vi "10-Tap 8-bit Camera without DRAM (FPGA-SIM).vi"() -> ()   [LabVIEW 2013]
doc: "This is the FPGA VI for the 10-Tap 8-Bit Camera with DRAM example. This example demonstrates how to acquire images from a 10-tap, 8-bit, extended configuration, Camera Link camera and transfer the images to the host. This example supports area scan and line scan cameras for both continuous and finite acquisitions.\n\nThis example also demonstrates the use of DRAM as a frame buffer for very high speed acquisitions. Data packing and flow-control are also employed to maximize use of the available DRAM and FIFOs in terms of both memory space and performance.\n\nAdditionally, the example demonstrates the serial server, which allows third-party camera configuration utilities to communicate with the camera using the Camera Link serial interface while this VI is running."
uses:
  Common/CL Signal Mapping.ctl
  Common/CL Configuration.ctl
  FPGA/Sector/Accumulate/Sector Parameter Cluster.ctl
  <vilib>/Platform/TimedLoop/XDataNode/timing_clust.ctl
  <vilib>/Platform/TimedLoop/XDataNode/nitl_modes.ctl
  <vilib>/Platform/TimedLoop/XDataNode/wakeup.ctl
  <vilib>/rvi/Emulation/niFpgaSctlEmulationGetInTimedLoop.vi
  <vilib>/rvi/Emulation/niFpgaEmulationReportErrorSimple.vi
  <vilib>/rvi/Emulation/niFpgaGetClockAttributes.vi
  <vilib>/rvi/Emulation/niFpgaCriticalErrorInLSC.vi
  <vilib>/rvi/FIFO/Fifo_Resource/nirvififoEmulationGetNumberOfElementsToWriteFpgaImpl.vi
  <vilib>/rvi/DataTransferAndStorage/Container/Common/niFpgaContainerGetUniqueNameForEmu.vi
  <vilib>/rvi/interface/RandomDataEmulation/nirviRandomDataFPGAFIFO.vi
  <vilib>/rvi/interface/RandomDataEmulation/niFpgaRandomDataHandleErrors.vi
  <vilib>/rvi/FIFO/Fifo_Resource/nirvififoEmulationWriteFpgaImpl.vi
  <vilib>/rvi/FIFO/Fifo_Resource/nirvififoEmulationGetNumberOfElementsToReadFpgaImpl.vi
  <vilib>/rvi/FIFO/Fifo_Resource/nirvififoEmulationReadFpgaImpl.vi
  <vilib>/rvi/Emulation/niFpgaProcessEmulError.vi
  FPGA/Globals/Sector Parameter Global.vi
  FPGA/Globals/Pixel Location Global.vi
  FPGA/Globals/Accumulated Sector Intensity.vi
  <vilib>/Platform/TimedLoop/XDataNode/XDataNode.xnode
  <vilib>/rvi/DataTransferAndStorage/Container/XNode/niFpgaContainer.xnode
  <vilib>/rvi/FIFO/Fifo_Resource/nirvififoEmulationGetNumberOfElementsToWrite.vi
  <vilib>/rvi/interface/RandomDataEmulation/nirviRandomDataFpgaReadWriteTemplate.vi
  <vilib>/rvi/FIFO/Fifo_Resource/nirvififoEmulationWrite.vi
  <vilib>/rvi/FIFO/Fifo_Resource/nirvififoEmulationGetNumberOfElementsToRead.vi
  <vilib>/rvi/FIFO/Fifo_Resource/nirvififoEmulationRead.vi
  <vilib>/Platform/TimedLoop/XDataNode/XDNodeRunTimeDep.lvlib
  FPGA/Globals/Wing Square Wave Frequency Global.vi
panel:
  out "Left Sector Edge":u8
  out "Right Sector Edge":u8
  in  "Right Start Angle Duty Cycle":fxp<+,8,0>
  in  "Right End Angle Duty Cycle":fxp<+,8,0>
  in  "Left End Angle Duty Cycle":fxp<+,8,0>
  in  "Left Start Angle Duty Cycle":fxp<+,8,0>
  out "Number of Elements to Write Sector Grouping FIFO":u32
  out "Analysis Ticks":u32
  out "Target Sim TO":bool
  out "Cam Data Timeout":bool
  out "Sector FIFO Timeout":bool
  out "Host DMA Timeout":bool
  out "Number of Elements to Read Cam Data":u32
  out "Number of Elements to Write Host DMA":u32
  in  "Words per image":u32=1000
  in  "Y Resolution":u16=1000
  in  "X Resolution":u16=1000
  in  "[Average BG Intensity]":u8[](array[numeric])=[0, 0, 0, 0, 0, 0, 0, 0, 0, 0, 0, 0, 0, 0, 0, 0, 0, 0, 0, 0, 0, 0, 0, 0, 0, 0, 0, 0, 0, 0, 0, 0]
  in  "Sector Threshold":u8
  in  "# of Frames to Average":u8=1
  in  "Sector Parameters Right":T1={"Start Angle"=0.0, "End Angle"=0.4708251953125, "Inner Radius"=309, "Outter Radius"=405, "Hinge X"=685, "Hinge Y"=527, "NumWingSectors"=8}
  in  "Sector Parameters Left":T1={"Start Angle"=0.65740966796875, "End Angle"=0.99468994140625, "Inner Radius"=309, "Outter Radius"=405, "Hinge X"=464, "Hinge Y"=534, "NumWingSectors"=8}
  in  "CL Config.Configuration":T2=enum."Full"
  in  "CL Config.Signal Mapping":T3=enum."Basler 10-tap"
  in  "CL Config.Line Scan":bool
  in  "CL Config.DVAL Active High":bool=TRUE
  in  "CL Config.LVAL Active High":bool=TRUE
  in  "CL Config.FVAL Active High":bool=TRUE
  in  "CL Config.Spare Active High":bool=TRUE
  in  "Acq Control.Line Scan Height":u32
  in  "Acq Control.Frames To Acq":u32
  in  "Acq Control.Acquire":bool
  in  "Acq Control.Cancel Acq":bool
  in  "Acq Control.Ignore DVAL":bool
  in  "Acq Control.Initialize":bool
  out "Acq Status.Acq In Progress":bool
  out "Acq Status.Clocks Per Line":u32
  out "Acq Status.Frames Acq'd":u32
  out "Acq Status.Lines Per Frame":u32
  out "Acq Status.DMA Write Timeout":bool
  out "Acq Status.Initialized":bool
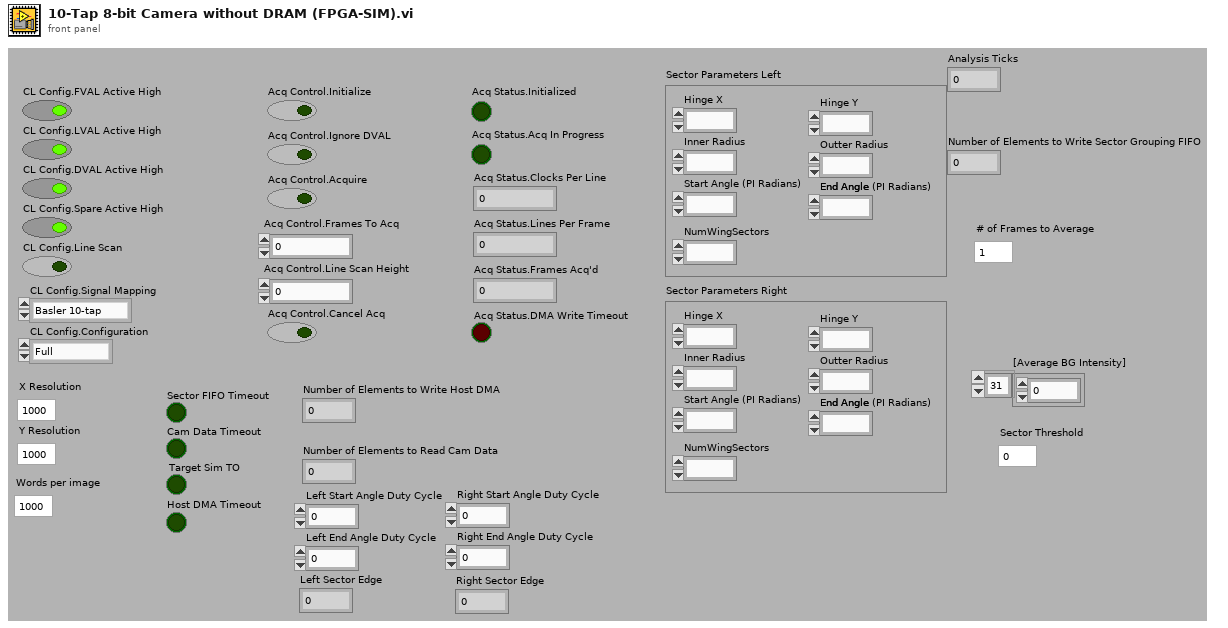
[diagram p1: front panel]
types:
  T1 = typedef "Sector Parameter Cluster.ctl" = cluster{"Start Angle":fxp<+/-,17,2>, "End Angle":fxp<+,17,3>, "Inner Radius":u16, "Outter Radius":u16, "Hinge X":u16, "Hinge Y":u16, "NumWingSectors":u8}
  T2 = typedef "CL Configuration.ctl" = enum8{"Base", "Medium", "Full"}
  T3 = typedef "CL Signal Mapping.ctl" = enum8{"Standard", "Basler 10-tap", "Vosskühler 10-tap"}
  T4 = typedef "XDNodeRunTimeDep.lvlib/timing_clust.ctl" = cluster{"Expected End [f-1]":u64, "Actual End [f-1]":u64, "Finished Late? [f-1]":bool, "Expected End [i-1]":u64, "Actual End [i-1]":u64, "Finished Late? [i-1]":bool, "Expected Start [i]":u64, "Actual Start [i]":u64, "Expected Start [f]":u64, "Actual Start [f]":u64, "Source Name":string, "Structure Name":string, "Period":i64, "Deadline":i64, "Offset":i64, "Start":i64, "Priority":i32, "Timeout":i32, "Mode":T5, "Wakeup Reason":T6, "Error":errorcluster, "Source Type":string, "Secondary Source Type":string, "Global End Time":u64, "Global Start Time":u64, "Frame Duration":u64, "Iteration Duration":u64, "Assigned CPU":i32, "I/O Scan Engine Mode":u32}
  T5 = typedef "XDNodeRunTimeDep.lvlib/nitl_modes.ctl" = enum32{"No Change", "Process missed periods, maintain original phase", "Discard missed periods, maintain original phase", "Process missed periods, ignore original phase", "Discard missed periods, ignore original phase"}
  T6 = typedef "XDNodeRunTimeDep.lvlib/wakeup.ctl" = enum32{"Normal", "Aborted", "Asynchronous wakeup", "Timing source error", "Timed loop error", "Timeout"}
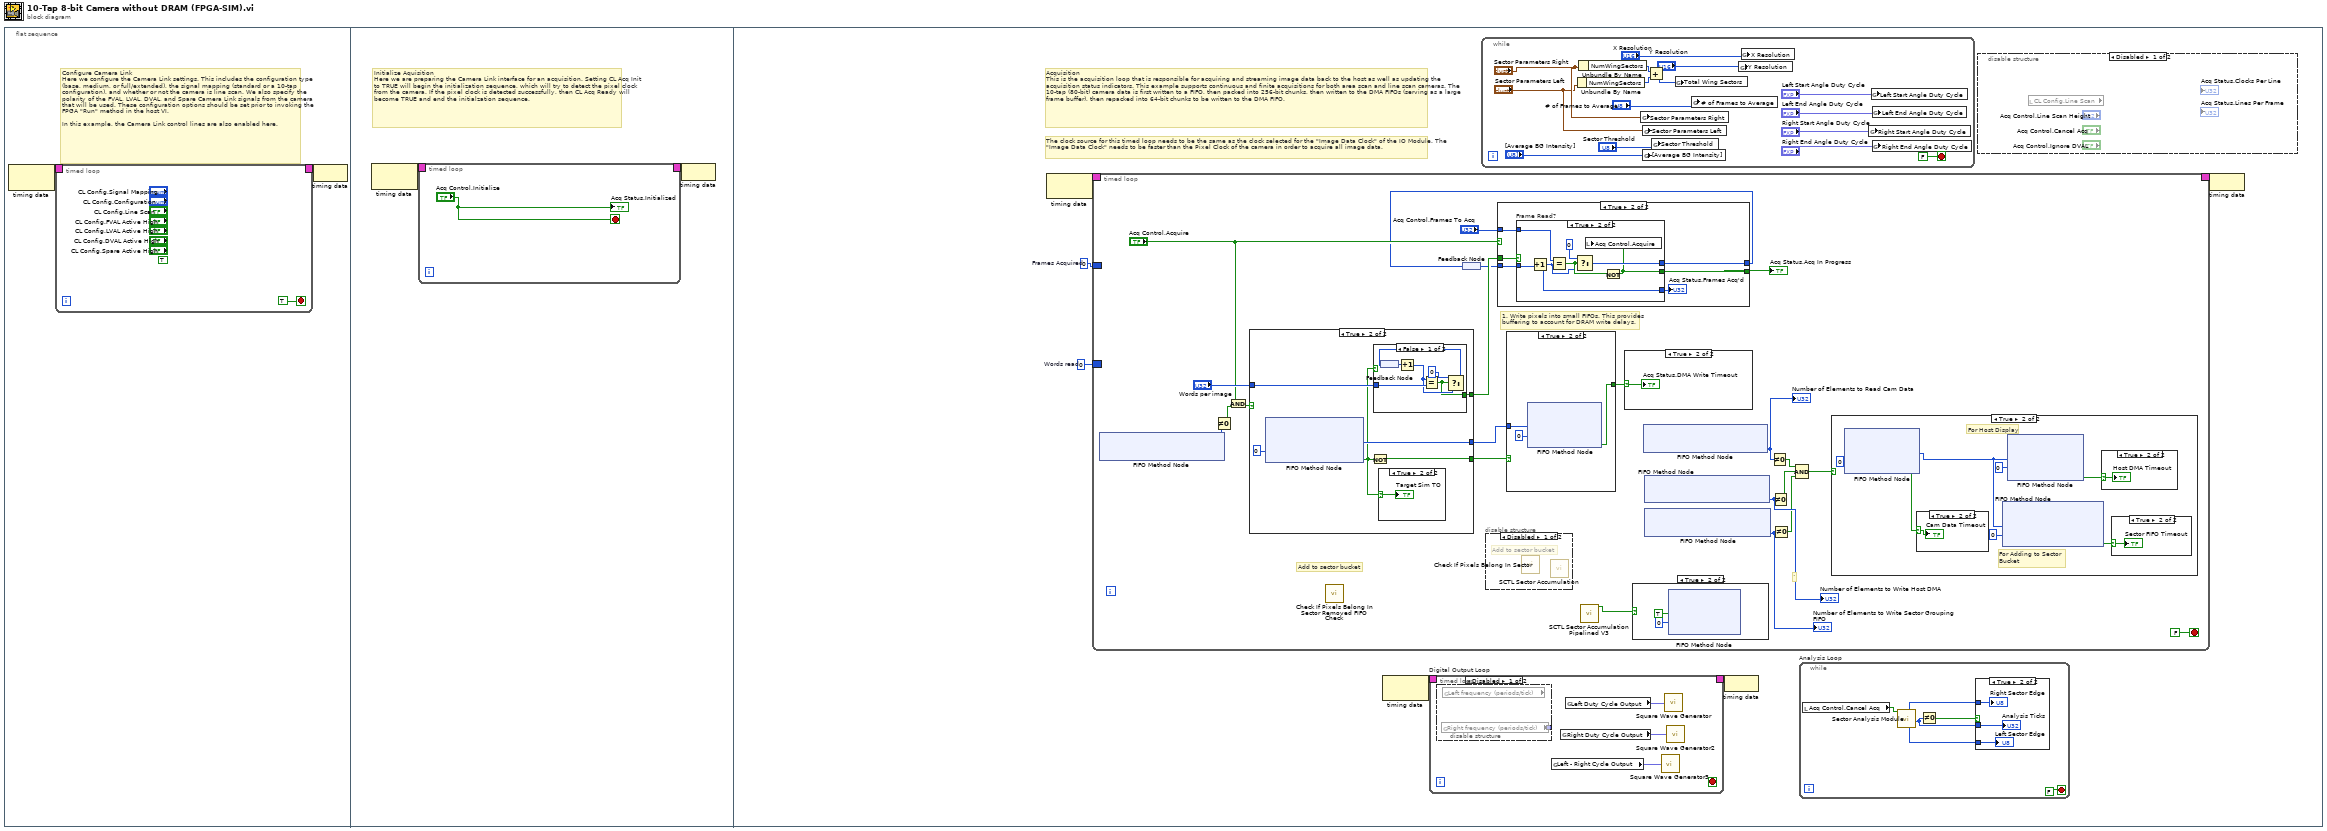
[diagram p0: block diagram]
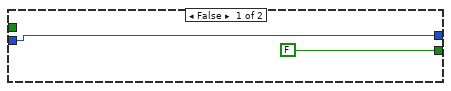
[diagram p8: hidden frame]
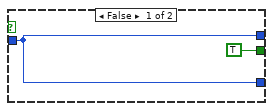
[diagram p9: hidden frame]
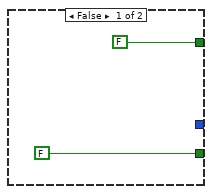
[diagram p10: hidden frame]
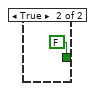
[diagram p12: hidden frame]
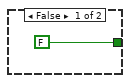
[diagram p17: hidden frame]
diagram:
  n1 = flat-sequence {
    frame #0 {
      # "Configure Camera Link\nHere we configure the Camera Link settings. This includes the configuration type (base, medium, or full/extended), the signal mapping (standard or a 10-tap configuration), and whether or not the camera is line scan. We also specify the polarity of the FVAL, LVAL, DVAL, and Spare Camera Link signals from the camera that will be used. These configuration options should be set prior to invoking the FPGA \"Run\" method in the host VI.\n\nIn this example, the Camera Link control lines are also enabled here."
      n2 = node-c288() -> (w2:T4)  [unwired: 1 in]
      n3 = timed-loop {
        timing: w2 -> [_]
        timing-out: [_] -> w1
        stop <- TRUE stop-if-true
        (unwired) TRUE ("IO Module\\CL Control Enable")
      }
      n4 = node-c288(w1) -> ()
    }
    frame #1 {
      # "Initialize Aquisition\nHere we are preparing the Camera Link interface for an acquisition. Setting CL Acq Init to TRUE will begin the initialization sequence, which will try to detect the pixel clock from the camera. If the pixel clock is detected successfully, then CL Acq Ready will become TRUE and end the initialzation sequence."
      n5 = node-c288() -> (w9:T4)  [unwired: 1 out]
      n6 = timed-loop {
        timing: w9 -> [_]
        timing-out: [_] -> w8
        stop <- "Acq Control.Initialize" stop-if-true
        "Acq Status.Initialized" <- "Acq Control.Initialize"
      }
      n7 = node-c288(w8) -> ()
    }
    frame #2 {
      w17 = u32 0  # Frames Acquired
      w18 = u32 0  # Words read
      # "The clock source for this timed loop needs to be the same as the clock selected for the \"Image Data Clock\" of the IO Module. The \"Image Data Clock\" needs to be faster than the Pixel Clock of the camera in order to acquire all image data."
      # "Acquisition\nThis is the acquisition loop that is responsible for acquiring and streaming image data back to the host as well as updating the acquisition status indicators. This example supports continuous and finite acquisitions for both area scan and line scan cameras. The 10-tap (80-bit) camera data is first written to a FIFO, then packed into 256-bit chunks, then written to the DMA FIFOs (serving as a large frame buffer), then repacked into 64-bit chunks to be written to the DMA FIFO."
      n8 = node-c288() -> (w20:T4)  [unwired: 1 in]
      n9 = timed-loop {
        timing: w20 -> [_]
        timing-out: [_] -> w19
        border: w18 -> [_]
        border: w17 -> [_]
        stop <- FALSE stop-if-true
        # "`"
        # "Add to sector bucket"
        # "1. Write pixels into small FIFOs. This provides\nbuffering to account for DRAM write delays."
        n10 = xnode ("FIFO Method Node")() -> ("Number of Elements to Write"=w53:u32)  [unwired: 1 in, 1 out]
        n11 = Not Equal To 0?(x=w53) -> (x != 0?=w52:bool)
        n12 = And(x="Acq Control.Acquire", y=w52) -> (x .and. y?=w60:bool)
        n13 = case shown="True" w60 {
          tunnel: [_ w92] -> w64
          tunnel: [FALSE w88] -> w62
          tunnel: "Words per image" -> [_ w90]
          tunnel: [FALSE w89] -> w49
          frame False {
          }
          frame True {
            n14 = xnode ("FIFO Method Node")("Timeout"=0) -> ("Element"=w92:u64, "Timed Out?"=w87:bool)  [unwired: 1 in, 1 out]
            n15 = Not(x=w87) -> (.not. x?=w88:bool)
            n16 = case shown="False" w87 {
              tunnel: w90 -> [w99 _]
              tunnel: [w94 FALSE] -> w89
              frame False {
                n17 = feedback #1() -> (w98:u32)
                n18 = Increment(x=w98) -> (x+1=w95:u32)
                n19 = Equal?(x=w95, y=w99) -> (x = y?=w94:bool)
                n20 = Select(t=u32 0 ("Acq Status.Frames Acq'd"), s=w94, f=w95) -> (s? t:f=w96:u32)
                n21 = feedback-in #1(w96) -> ()
              }
              frame True {
              }
            }
            n22 = case shown="True" w87 {
              selector: w87 -> [_ w93]
              frame False {
              }
              frame True {
                "Target Sim TO" <- w93
              }
            }
          }
        }
        n23 = call "Check If Pixels Belong In Sector Removed FIFO Check.vi"() -> ()  [unwired: 11 in, 1 out]
        n24 = feedback #2() -> (w48:u32)
        n25 = disable-structure shown="Disabled" {
          frame Disabled {
            # "Add to sector bucket"
            n26 = call "Check If Pixels Belong In Sector.vi"() -> ()  [unwired: 11 in, 1 out]
            n27 = call "SCTL Sector Accumulation.vi"() -> ()  [unwired: 11 in, 1 out]
          }
          frame Enabled {
          }
        }
        n28 = case shown="True" "Acq Control.Acquire" {
          tunnel: w49 -> [_ w75]
          tunnel: w48 -> [w69 w74]
          tunnel: "Acq Control.Frames To Acq" -> [_ w73]
          tunnel: [w69 w72] -> w46
          tunnel: [FALSE w71] -> w45
          frame False {
          }
          frame True {
            n29 = case "Frame Read?" shown="True" w75 {
              tunnel: w74 -> [w76 w84]
              tunnel: w73 -> [_ w83]
              tunnel: [w76 w81] -> w72
              tunnel: [TRUE w79] -> w71
              tunnel: [w76 w78] -> w70
              frame False {
              }
              frame True {
                n30 = Increment(x=w84) -> (x+1=w78:u32)
                n31 = Equal?(x=w83, y=w78) -> (x = y?=w80:bool)
                n32 = Select(t=u32 0 ("Frames Acquired"), s=w80, f=w78) -> (s? t:f=w81:u32)
                n33 = Not(x=w80) -> (.not. x?=w79:bool)
                n34 = local write "Acq Control.Acquire"(w79) -> ()
              }
            }
            "Acq Status.Frames Acq'd" <- w70
          }
        }
        "Acq Status.Acq In Progress" <- w45
        n35 = feedback-in #2(w46) -> ()
        n36 = case shown="True" w62 {
          tunnel: [FALSE ("Timed Out?") w113] -> w44
          tunnel: w64 -> [_ w114]
          frame False {
          }
          frame True {
            n37 = xnode ("FIFO Method Node")("Element"=w114, "Timeout"=0) -> ("Timed Out?"=w113:bool)  [unwired: 1 in, 1 out]
          }
        }
        n38 = call "SCTL Sector Accumulation Pipelined V3.vi"() -> ("New Data?"=w43:bool)  [unwired: 11 in]
        n39 = case shown="True" w44 {
          selector: w44 -> [_ w67]
          frame False {
          }
          frame True {
            "Acq Status.DMA Write Timeout" <- w67
          }
        }
        n40 = case shown="True" w43 {
          frame False {
          }
          frame True {
            n41 = xnode ("FIFO Method Node")("Element"=TRUE, "Timeout"=0) -> ()  [unwired: 1 in, 2 out]
          }
        }
        n42 = xnode ("FIFO Method Node")() -> ("Number of Elements to Read"=w55:u32)  [unwired: 1 in, 1 out]
        "Number of Elements to Read Cam Data" <- w55
        n43 = xnode ("FIFO Method Node")() -> ("Number of Elements to Write"=w58:u32)  [unwired: 1 in, 1 out]
        "Number of Elements to Write Host DMA" <- w58
        n44 = xnode ("FIFO Method Node")() -> ("Number of Elements to Write"=w57:u32)  [unwired: 1 in, 1 out]
        "Number of Elements to Write Sector Grouping FIFO" <- w57
        n45 = Not Equal To 0?(x=w55) -> (x != 0?=w54:bool)
        n46 = Not Equal To 0?(x=w58) -> (x != 0?=w59:bool)
        n47 = Not Equal To 0?(x=w57) -> (x != 0?=w56:bool)
        n48 = Compound Arithmetic op=AND(w54, w59, w56) -> (w61:bool)
        n49 = case shown="True" w61 {
          frame False {
          }
          frame True {
            # "For Adding to Sector \nBucket"
            # "For Host Display"
            n50 = xnode ("FIFO Method Node")("Timeout"=0) -> ("Element"=w105:u64, "Timed Out?"=w101:bool)  [unwired: 1 in, 1 out]
            n51 = case shown="True" w101 {
              selector: w101 -> [_ w108]
              frame False {
              }
              frame True {
                "Cam Data Timeout" <- w108
              }
            }
            n52 = xnode ("FIFO Method Node")("Element"=w105, "Timeout"=0) -> ("Timed Out?"=w103:bool)  [unwired: 1 in, 1 out]
            n53 = xnode ("FIFO Method Node")("Element"=w105, "Timeout"=0) -> ("Timed Out?"=w102:bool)  [unwired: 1 in, 1 out]
            n54 = case shown="True" w102 {
              selector: w102 -> [_ w109]
              frame False {
              }
              frame True {
                "Host DMA Timeout" <- w109
              }
            }
            n55 = case shown="True" w103 {
              selector: w103 -> [_ w110]
              frame False {
              }
              frame True {
                "Sector FIFO Timeout" <- w110
              }
            }
          }
        }
      }
      n56 = node-c288() -> (w16:T4)  [unwired: 1 in]
      n57 = timed-loop "Digital Output Loop" {
        timing: w16 -> [_]
        timing-out: [_] -> w15
        stop <- _ stop-if-true
        n58 = disable-structure shown="Disabled" {
          disable-tunnel: [w24 _] -> _
          frame Disabled {
            n59 = global read "Wing Square Wave Frequency Global.vi" "Right frequency (periods/tick)"() -> (w24:fxp<+,32,0>)
            n60 = global read "Wing Square Wave Frequency Global.vi" "Left frequency (periods/tick)"() -> ()  [unwired: 1 out]
          }
          frame Enabled {
          }
        }
        n61 = global read "Sector Parameter Global.vi" "Left - Right Cycle Output"() -> (w21:fxp<+,8,0>)
        n62 = global read "Sector Parameter Global.vi" "Right Duty Cycle Output"() -> (w22:fxp<+,8,0>)
        n63 = global read "Sector Parameter Global.vi" "Left Duty Cycle Output"() -> (w23:fxp<+,8,0>)
        n64 = call "Square Wave Generator3"("duty cycle (periods)"=w21) -> ()  [unwired: 14 in, 1 out]
        n65 = call "Square Wave Generator"("duty cycle (periods)"=w23) -> ()  [unwired: 14 in, 1 out]
        n66 = call "Square Wave Generator2"("duty cycle (periods)"=w22) -> ()  [unwired: 14 in, 1 out]
      }
      n67 = while {
        stop <- FALSE stop-if-true
        n68 = Unbundle By Name("Sector Parameters Left") -> ("NumWingSectors"=w131:u8)
        n69 = Unbundle By Name("Sector Parameters Right") -> ("NumWingSectors"=w132:u8)
        n70 = global write "Sector Parameter Global.vi" "Sector Parameters Right"("Sector Parameters Right") -> ()
        n71 = global write "Sector Parameter Global.vi" "Sector Parameters Left"("Sector Parameters Left") -> ()
        n72 = global write "Sector Parameter Global.vi" "[Average BG Intensity]"("[Average BG Intensity]") -> ()
        n73 = Add(x=w132, y=w131) -> (x+y=w130:u8)
        n74 = global write "Sector Parameter Global.vi" "Sector Threshold"("Sector Threshold") -> ()
        n75 = global write "Accumulated Sector Intensity.vi" "Total Wing Sectors"(w130) -> ()
        n76 = global write "Pixel Location Global.vi" "# of Frames to Average"("# of Frames to Average") -> ()
        n77 = global write "Pixel Location Global.vi" "Y Resolution"("Y Resolution") -> ()
        n78 = global write "Pixel Location Global.vi" "X Resolution"("X Resolution") -> ()
        n79 = global write "Sector Parameter Global.vi" "Right Start Angle Duty Cycle"("Right Start Angle Duty Cycle") -> ()
        n80 = global write "Sector Parameter Global.vi" "Left Start Angle Duty Cycle"("Left Start Angle Duty Cycle") -> ()
        n81 = global write "Sector Parameter Global.vi" "Left End Angle Duty Cycle"("Left End Angle Duty Cycle") -> ()
        n82 = global write "Sector Parameter Global.vi" "Right End Angle Duty Cycle"("Right End Angle Duty Cycle") -> ()
      }
      n83 = node-c288(w15) -> ()
      n84 = while "Analysis Loop" {
        stop <- FALSE stop-if-true
        n85 = local read "Acq Control.Cancel Acq"() -> (w38:bool)
        n86 = call "Sector Analysis Module.vi"("Canceled?"=w38) -> ("Analysis Ticks"=w37:u32, "Left Sector Edge"=w34:u8, "Right Sector Edge"=w35:u8)  [unwired: 6 in, 2 out]
        n87 = Not Equal To 0?(x=w37) -> (x != 0?=w36:bool)
        n88 = case shown="True" w36 {
          tunnel: w37 -> [_ w42]
          tunnel: w35 -> [_ w41]
          tunnel: w34 -> [_ w40]
          frame False {
          }
          frame True {
            "Analysis Ticks" <- w42
            "Right Sector Edge" <- w41
            "Left Sector Edge" <- w40
          }
        }
      }
      n89 = disable-structure shown="Disabled" {
        frame Disabled {
          n90 = local read "CL Config.Line Scan"() -> (w31:bool)
        }
        frame Enabled {
        }
      }
      n91 = node-c288(w19) -> ()
    }
  }
